vi "SOUR_POW_ATT.vi"(0 "VISA IN":refnum<visa-resource-name>, 4 "Atten(db)":dbl=10.0, 5 "error in":errorcluster, 7 "Channel":i32=1, 9 "Port":i32=1) -> (14 "VISA Out":refnum<visa-resource-name>, 19 "error out":errorcluster)   [LabVIEW 2018, in "PNA-X.lvlib"]
doc: "SOURce:POWer:ATTenuation <num>. \n[src] String. (NOT case sensitive). Source port. Optional. Use SOUR:CAT? to \nreturn a list of valid port names. \nWhile this argument can be used to make settings for ALL ports, it is designed \nto access ports that are not simple numbers, such as \"Port 1 Src2\". Otherwise, \nthe <port> argument performs the same function. If both arguments are \nspecified, [src] takes priority. \nExamples SOUR:POW2:ATT:Auto On \nsource2:power:attentuation:auto off \nsour:pow:att:auto 1, \"Port 1 Src2\" \nQuery Syntax SOURce<cnum>:POWer:ATTenuation:Auto? [src] \nReturn Type Boolean (1 = ON, 0 = OFF) \nDefault ON \nSOURce<cnum>:POWer:CENTer <num> \n1827\n\n(Read-Write) Sets the power sweep center power. Must also set: \nSENS:SWE:TYPE POWer and SOURce:POWer:SPAN <num>. \nParameters \n<cnum> Any existing channel number. If unspecified, value is set to 1 \n<num> Center power. Actual achievable leveled power depends on frequency. \nExamples SOUR:POW:CENT -15 \nsource2:power:center -7 \nQuery Syntax SOURce<cnum>:POWer:CENTer? \nReturn Type Numeric \nDefault 0 dBm \nSOURce<cnum>:POWer:COUPle <ON | OFF> \n(Read-Write) Turns Port Power Coupling ON or OFF. \nParameters \n<cnum> Any existing channel number. If unspecified, value is set to 1 \n<ON | OFF> ON (or 1) - turns coupling ON. The same power level is used for both source \nports. \nOFF (or 0) - turns coupling OFF. Power level can be set individually for each \nsource port. \nExamples SOUR:POW:COUP ON \nsource2:power:couple off \nQuery Syntax SOURce<cnum>:POWer:COUPle? \nReturn Type Boolean (1 = ON, 0 = OFF) \nDefault ON \nSOURce<cnum>:POWer:DETector <char> OBSOLETE \n1828\n\n(Read-Write) The PNA models with external leveling are now OBSOLETE. \nSets the source leveling loop as Internal or External. \nParameters \n<cnum> Any existing channel number. If unspecified, value is set to 1 \n<char> INTernal - Internal leveling is applied to the source \nEXTernal - External leveling is applied to the source through a rear-panel \nconnector. ONLY provided on 3 GHz, 6 GHz, and 9 GHz PNA models. \nExamples SOUR:POW:DET INT \nsource2:power:detector external \nQuery Syntax SOURce<cnum>:POWer:DETector? \nReturn Type Character \nDefault INTernal \nSOURce<cnum>:POWer<port>[:LEVel][:IMMediate] \n[:AMPLitude] <num>, [src] \n(Read-Write) Sets the RF power output level. \nParameters \n<cnum> Any existing channel number. If unspecified, value is set to 1 \n<port> Port number of the PNA. If unspecified, value is set to 1. To make settings for \nports that are not simple numbers, use the [src] argument. \n<num> Source power in dBm. \nNote: The range of settable power values depends on the PNA model and if \nsource attenuators are installed. To determine the range of values, perform a \nquery using MAX, then MIN, as an argument. (SOUR:POW:ATT:AUTO must \nbe set to ON) Example: SOURce:POWer? Max \nActual achievable leveled power depends on frequency. \n[src] String. (NOT case sensitive). Source port. Optional. Use SOUR:CAT? to \nreturn a list of valid port names. \nWhile this argument can be used to make settings for ALL ports, it is designed \nto access ports that are not simple numbers, such as \"Port 1 Src2\". Otherwise, \nthe <port> argument performs the same function. If both arguments are \nspecified, [src] takes priority.\n1829\n\nExamples SOUR:POW1 5DB \nsource2:power:level:immediate:amplitude maximum \nsour:pow 5, \"Port 1 Src2\" \nQuery Syntax SOURce<cnum>:POWer[:LEVel][:IMMediate][:AMPLitude]? [src] \nReturn Type Numeric \nDefault 0 dBm \nSOURce<cnum>:POWer[:LEVel]:SLOPe <num> \n(Read-Write) Sets the RF power slope value. \nParameters \n<cnum> Any existing channel number. If unspecified, value is set to 1 \n<num> Slope value in db/GHz. Choose any integer between -2 and 2 (0 is no slope). \nExamples SOUR:POW:SLOP 2 \nsource2:power:slope -2 \nQuery Syntax SOURce<cnum>:POWer[:LEVel]:SLOPe? \nReturn Type Numeric \nDefault 0 \nSOURce<cnum>:POWer[:LEVel]:SLOPe:STATe <ON | OFF> \n(Read-Write) Turns Power Slope ON or OFF. \nParameters \n<cnum> Any existing channel number. If unspecified, value is set to 1 \n<ON|OFF> ON (or 1) - turns slope ON. \nOFF (or 0) - turns slope OFF. \nExamples SOUR:POW:SLOP:STAT ON \nsource2:power:slope:state off \nQuery Syntax SOURce<cnum>:POWer[:LEVel]:SLOPe:STATe? \nReturn Type Boolean (1 = ON, 0 = OFF) \nDefault OFF \nSOURce<cnum>:POWer<port>:MODE <state>, [src] \n1830\n\n(Read-Write) Sets the state of PNA source for the specified port. \nLearn more about the PNA internal second source \nParameters \n<cnum> Any existing channel number. If unspecified, value is set to 1 \n<port> Port number of the PNA. If unspecified, <port> is set to 1. To make settings for \nports that are not simple numbers, use the [src] argument. \n<state> Source state. Choose from: \nAUTO Source power is turned ON when required for a measurement. \nON Source power is always ON regardless of the measurement. \nOFF Source power is always OFF regardless of the measurement. \nNote: ON and OFF are valid only on PNA models with two sources. \n[src] String. (NOT case sensitive). Source port. Optional. Use SOUR:CAT? to \nreturn a list of valid port names. \nWhile this argument can be used to make settings for ALL ports, it is designed \nto access ports that are not simple numbers, such as \"Port 1 Src2\". Otherwise, \nthe <port> argument performs the same function. If both arguments are \nspecified, [src] takes priority. \nExamples SOUR:POW:MODE ON \nsource2:power4:mode OFF \nsour:pow:mode 1, \"Port 1 Src2\" \nQuery Syntax SOURce<cnum>:POWer<port>:MODE? [src} \nReturn Type Character \nDefault Auto \nSOURce<cnum>:POWer:SPAN <num> \n1831\n\n(Read-Write) Sets the power sweep span power. Must also set: \nSENS:SWE:TYPE POWer and SOURce:POWer:CENTer <num>. \nParameters \n<cnum> Any existing channel number. If unspecified, value is set to 1. \n<num> Span power. Actual achievable leveled power depends on frequency. \nExamples SOUR:POW:SPAN -15 \nsource2:power:span -7 \nQuery Syntax SOURce<cnum>:POWer:SPAN? \nReturn Type Numeric \nDefault 0 dBm \nSOURce<cnum>:POWer:STARt <num> \n(Read-Write) Sets the power sweep start power. Must also set \nSENS:SWE:TYPE POWer and SOURce:POWer:STOP <num>. \nParameters \n<cnum> Any existing channel number. If unspecified, value is set to 1 \n<num> Start power. \nNote: The range of settable power values depends on the PNA model and if \nsource attenuators are installed. To determine the range of values, perform a \nquery using MAX, then MIN, as an argument. (SOUR:POW:ATT:AUTO must \nbe set to ON) Example: SOURce:POWer:STARt? MIN \nActual achievable leveled power depends on frequency. \nExamples SOUR:POW:STAR -15 \nsource2:power:start -7 \nQuery Syntax SOURce<cnum>:POWer:STARt? \nReturn Type Numeric \nDefault 0 dBm \nSOURce<cnum>:POWer:STOP <num> \n1832\n\n(Read-Write) Sets the power sweep stop power. Must also set: SENS:SWE:TYPE POWer and"
uses:
  PNA-X.lvlib
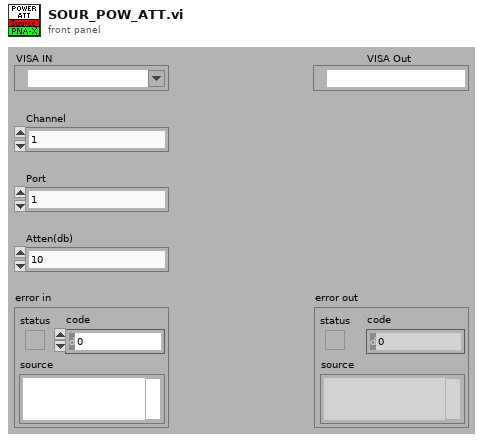
[diagram p1: front panel]
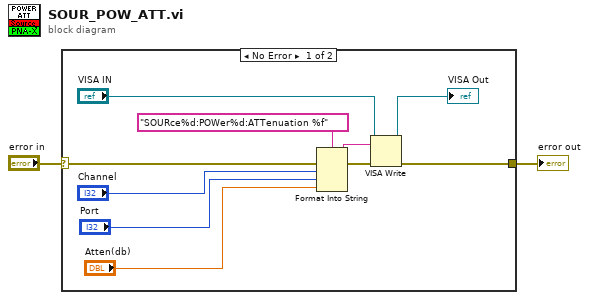
[diagram p0: block diagram]
diagram:
  n1 = case shown="No Error" "error in" {
    selector: "error in" -> [w12 w13]
    tunnel: [w7 w13] -> w1
    frame No Error {
      n2 = Format Into String(format string="SOURce%d:POWer%d:ATTenuation %f" ("Cmdline"), error in=w12, "Channel", "Port", "Atten(db)") -> (resulting string=w10:string, error out=w11:errorcluster)  [unwired: 1 in]
      n3 = VISA Write(VISA resource name="VISA IN", write buffer=w10, error in (no error)=w11) -> (VISA resource name out=→"VISA Out":refnum<visa-resource-name>, error out=w7:errorcluster)  [unwired: 1 out]
    }
    frame Error {
    }
  }
  "error out" <- w1
